vi "R5_Setup.vi"() -> (1 "tdms file out":refnum<k34>, 2 "error out":errorcluster)   [LabVIEW 2016]
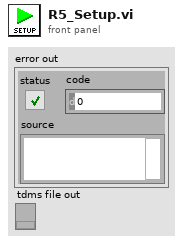
[diagram p1: front panel]
types:
  T1 = enum16{"open", "open or create", "create or replace", "create", "open (read-only)"}
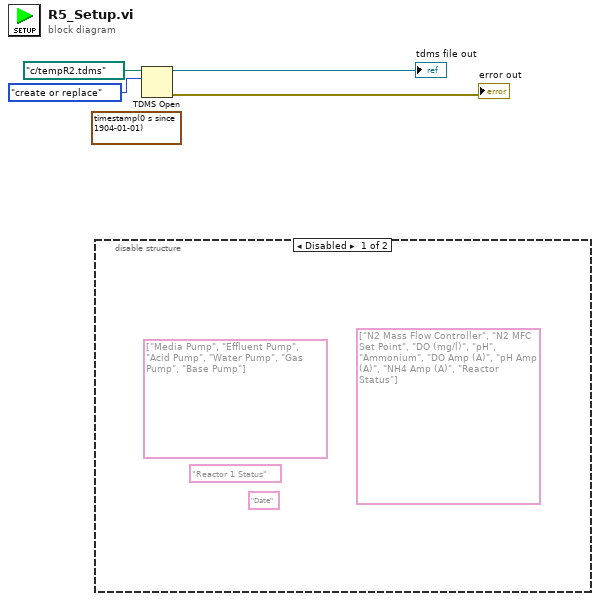
[diagram p0: block diagram]
diagram:
  (unwired) timestamp(0 s since 1904-01-01)
  n1 = disable-structure shown="Disabled" {
    frame Disabled {
      (unwired) string[] ["N2 Mass Flow Controller", "N2 MFC Set Point", "DO (mg/l)", "pH", "Ammonium", "DO Amp (A)", "pH Amp (A)", "NH4 Amp (A)", "Reactor Status"] ("channel name(s)")
      (unwired) string[] ["Media Pump", "Effluent Pump", "Acid Pump", "Water Pump", "Gas Pump", "Base Pump"] ("channel name(s)")
      (unwired) "Date" ("group name in (Untitled)")
      (unwired) "Reactor 1 Status" ("group name in (Untitled)")
    }
    frame Enabled {
    }
  }
  n2 = TDMS Open(10:T1."create or replace" ("operation (0:open)"), 11:path "c:/tempR2.tdms" ("file path")) -> (0:→"error out":errorcluster, 3:→"tdms file out":refnum<k34>)  [unwired: 5 in]
